vi "Get Plugins Root Path.vi"(0 "error in (no error)":errorcluster) -> (3 "plugins root path":path, 8 "error out":errorcluster)   [LabVIEW 2024, in "SEECD System Explorer.lvlib"]
uses:
  SEECD System Explorer.lvlib
  NationalInstruments.VeriStand
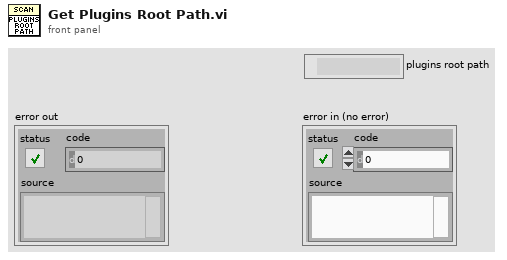
[diagram p1: front panel]
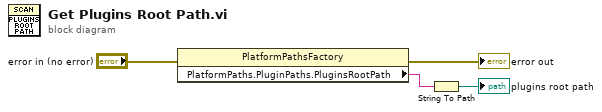
[diagram p0: block diagram]
diagram:
  n1 = property class="PlatformPathsFactory"(error in="error in (no error)") -> (error out=→"error out":errorcluster, "PlatformPaths.PluginPaths.PluginsRootPath"=w1:string)  [unwired: 1 in, 1 out]
  n2 = String To Path(string=w1) -> (path=→"plugins root path":path)
